vi "Trajectory_boom.vi"(0 "i":i32, 1 "if p2p":bool, 2 "ifSin?":bool, 3 "Target_Angle":dbl, 4 "if end8":bool, 5 "q":dbl[](array[numeric]), 7 "qd":dbl[](array[numeric]), 9 "qdd":dbl[](array[numeric]), 10 "if  Ramp":bool, 11 "qddd":dbl[](array[numeric]), 12 "qd8_1":dbl[](array[numeric]), 13 "qd8_dot_2":dbl[](array[numeric]), 14 "qd8_ddot_2":dbl[](array[numeric])) -> (6 "qd1_tol":dbl[](array[numeric]))   [LabVIEW 2020]
uses:
  <vilib>/imath/engines/lvmath2/RunTimeEngine/Managers/WorkSpace/UID Generator.vi
  <vilib>/imath/engines/lvmath2/RunTimeEngine/RunTimeType/NIMS_RunTimeType_From StrictType (excl LVString).vi
  <instcachedir>/0/NIMS_RunTimeType_From StrictType (excl LVString)_283B1B2000484AAA8744D21CE97EA49F.lvgen/NIMS_RunTimeType_From StrictType (excl LVString)_283B1B2000484AAA8744D21CE97EA49F_000.vi
  <vilib>/imath/engines/lvmath2/RunTimeEngine/LocalVariableDefStatement/MC_LocalVariableDefStatement_Display.vi
  <vilib>/imath/engines/lvmath2/RunTimeEngine/Managers/SymbolTable/Clear UID.vi
  <vilib>/imath/engines/lvmath2/RunTimeEngine/NodeEndStatement/NIMS_NodeEndStatement_Output.vi
  <instcachedir>/0/NIMS_NodeEndStatement_Output_53EC0D466D134D7ABD903AC30B43404B.lvgen/NIMS_NodeEndStatement_Output_53EC0D466D134D7ABD903AC30B43404B_001.vi
  <vilib>/imath/engines/lvmath2/RunTimeEngine/ErrorHandling/NIMS_Finalize Error.vi
  <vilib>/imath/engines/lvmath2/RunTimeEngine/VariableToken/NIMS_VariableToken_CondDefined.vi
  <instcachedir>/0/NIMS_VariableToken_CondDefined_537E119D71C74F9D9452D6FF923F1E1F.lvgen/NIMS_VariableToken_CondDefined_537E119D71C74F9D9452D6FF923F1E1F_003.vi
  <vilib>/imathl/engines/lvmath/Functions/Error Handling/Create Error.vi
  <instcachedir>/0/NIMS_VariableToken_CondDefined_537E119D71C74F9D9452D6FF923F1E1F.lvgen/NIMS_VariableToken_CondDefined_537E119D71C74F9D9452D6FF923F1E1F_005.vi
  <vilib>/imath/engines/lvmath/Functions/Error Handling/MergeErrorsWrapper.vi
  <instcachedir>/0/NIMS_NodeEndStatement_Output_53EC0D466D134D7ABD903AC30B43404B.lvgen/NIMS_NodeEndStatement_Output_53EC0D466D134D7ABD903AC30B43404B_010.vi
  <instcachedir>/0/NIMS_NodeEndStatement_Output_53EC0D466D134D7ABD903AC30B43404B.lvgen/NIMS_NodeEndStatement_Output_53EC0D466D134D7ABD903AC30B43404B_005.vi
  <vilib>/imath/engines/lvmath2/RunTimeEngine/Managers/SymbolTable/NIMS_WorkSpace.lvlib
panel:
  out "AlphaWF":dbl
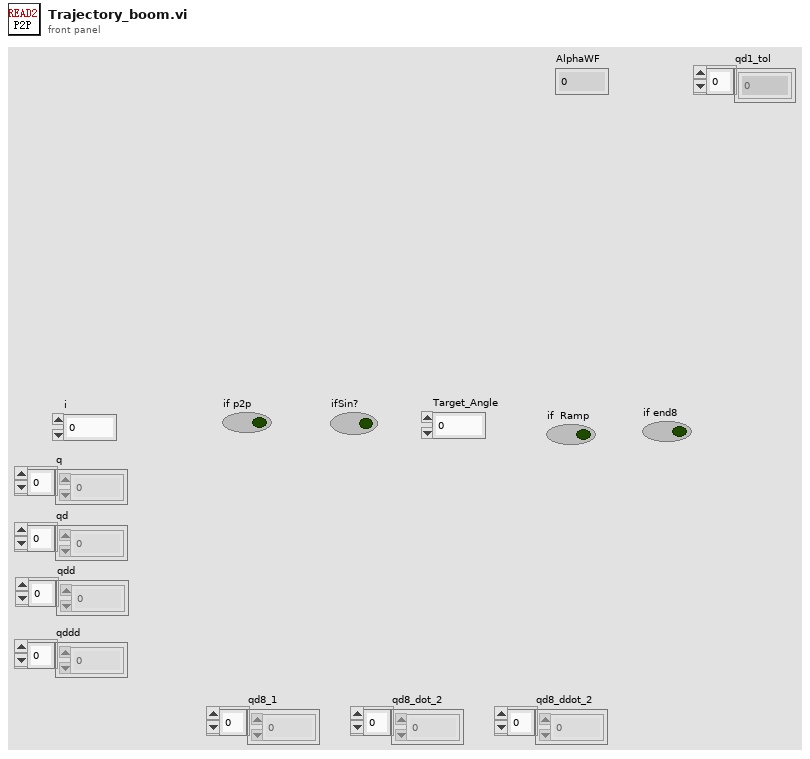
[diagram p1: front panel]
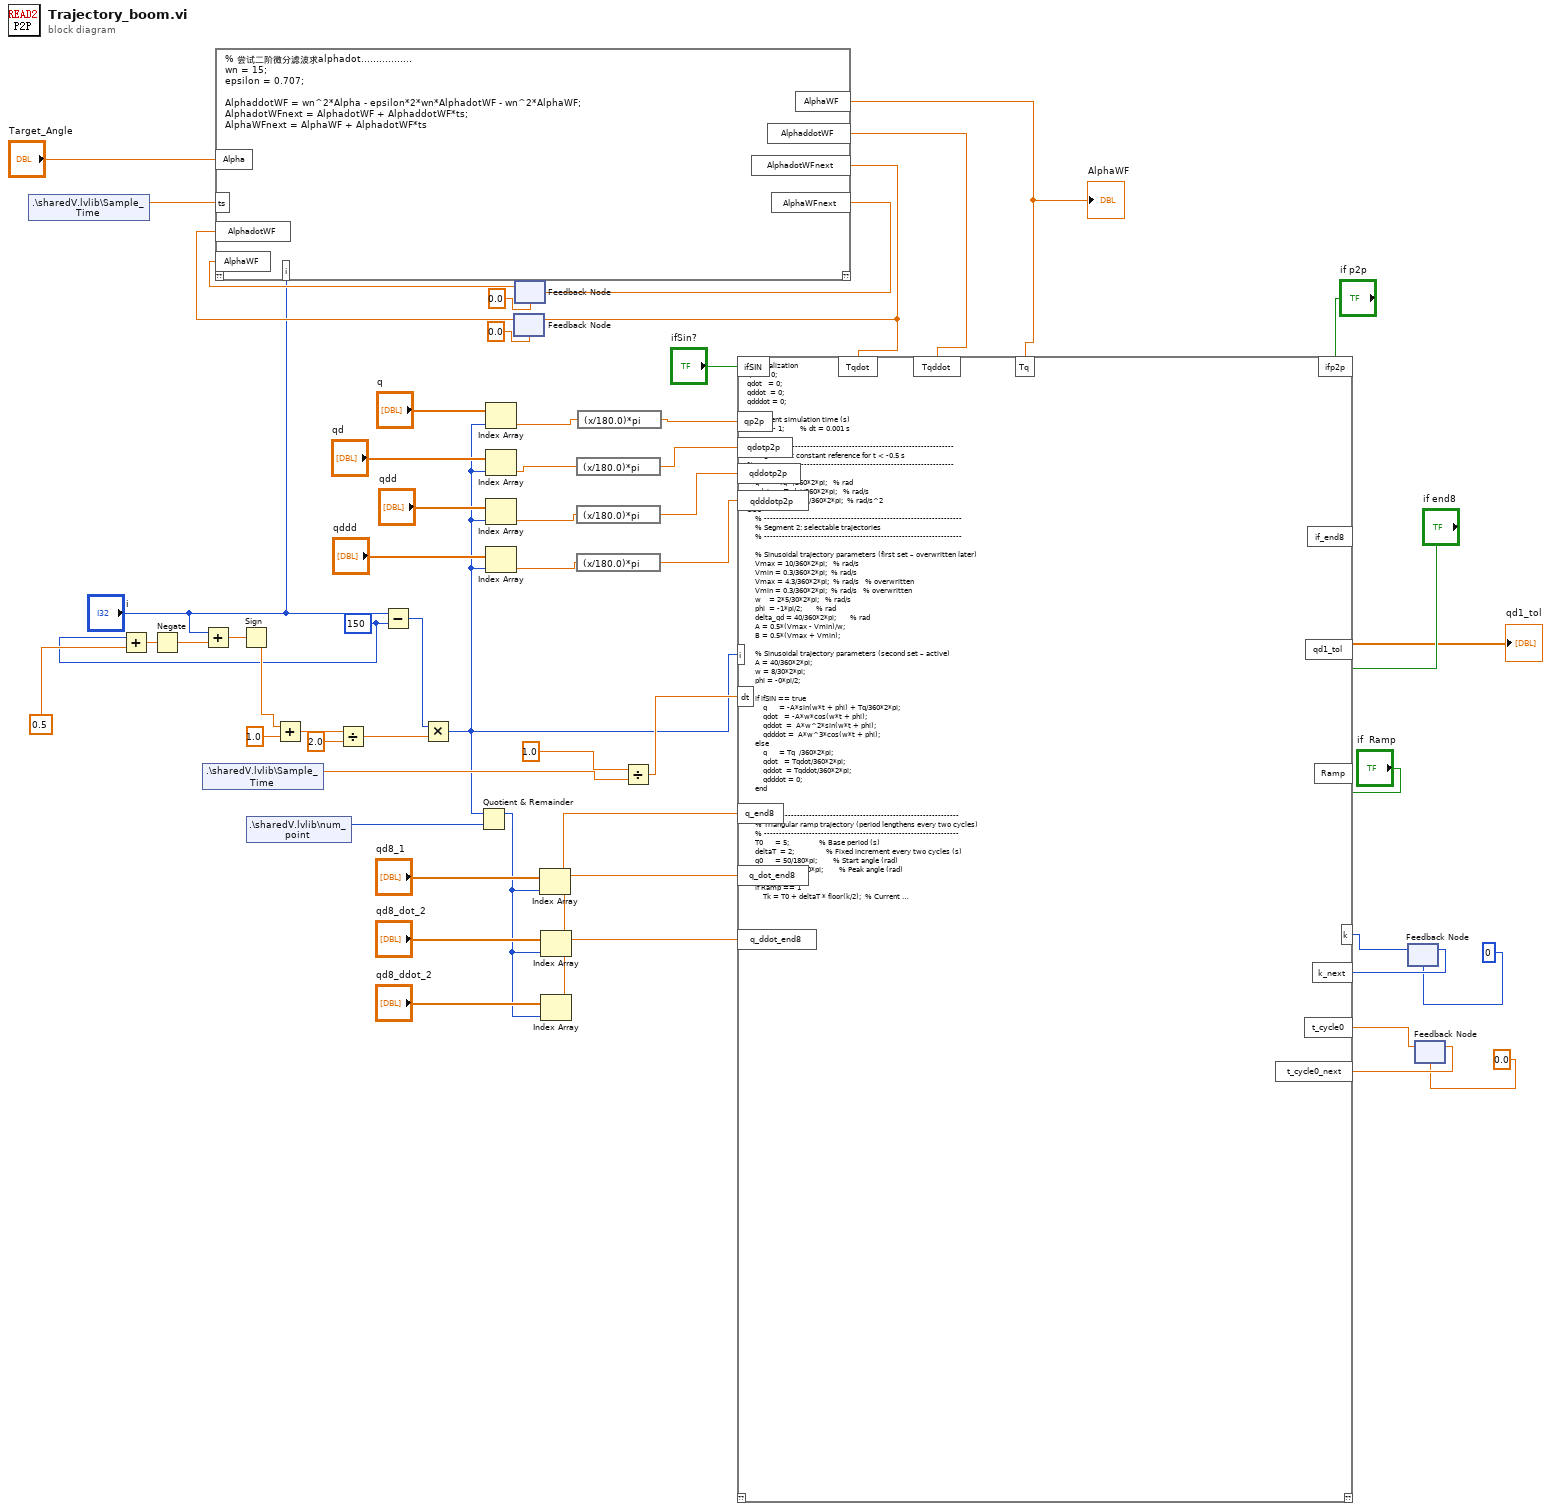
[diagram p0: block diagram]
diagram:
  w31 = 150 ("y")
  n1 = shared-variable ".\\sharedV.lvlib\\Sample_Time"() -> (w45:dbl)  [unwired: 1 in, 1 out]
  n2 = Add(x=w31, y=0.5) -> (x+y=w32:dbl)
  n3 = Negate(x=w32) -> (-x=w41:dbl)
  n4 = Add(x="i", y=w41) -> (x+y=w40:dbl)
  n5 = shared-variable ".\\sharedV.lvlib\\Sample_Time"() -> (w43:dbl)  [unwired: 1 in, 1 out]
  n6 = Sign(1:w40) -> (0:w38:dbl)
  n7 = shared-variable ".\\sharedV.lvlib\\num_point"() -> (w23:i32)  [unwired: 1 in, 1 out]
  n8 = Add(x=w38, y=1.0) -> (x+y=w36:dbl)
  n9 = Divide(x=w36, y=2.0) -> (x/y=w35:dbl)
  n10 = Subtract(x="i", y=w31) -> (x-y=w34:i32)
  n11 = Multiply(x=w34, y=w35) -> (x*y=w20:i32)
  n12 = Quotient & Remainder(x=w20, y=w23) -> (x-y*floor(x/y)=w22:i32)  [unwired: 1 out]
  n13 = Index Array(array="q", index=w20) -> (element=w12:dbl)
  n14 = Index Array(array="qd", index=w20) -> (element=w14:dbl)
  n15 = Index Array(array="qdd", index=w20) -> (element=w17:dbl)
  n16 = Index Array(array="qddd", index=w20) -> (element=w18:dbl)
  n17 = feedback #1(0.0 ("AlphadotWFnext")) -> (w47:dbl)
  n18 = feedback #2(0.0 ("AlphaWFnext")) -> (w49:dbl)
  n19 = mathscript code="% 尝试二阶微分滤波求alphadot.................\nwn = 15;\nepsilon = 0.707;\n\nAlphaddotWF = wn^2*Alpha - epsilon*2*wn*AlphadotWF - wn^2*AlphaWF;\nAlphadotWFnext = AlphadotWF + AlphaddotWF*ts;\nAlphaWFnext = AlphaWF + AlphadotWF*ts"("AlphaWF"=w49, "ts"=w45, "AlphadotWF"=w47, "Alpha"="Target_Angle", "i"="i") -> ("AlphaWFnext"=w50:dbl, "AlphadotWFnext"=w8:dbl, "AlphaWF"=w10:dbl, "AlphaddotWF"=w9:dbl)  [unwired: 1 in, 1 out]
  "AlphaWF" <- w10
  n20 = feedback-in #1(w8) -> ()
  n21 = feedback-in #2(w50) -> ()
  n22 = Index Array(array="qd8_1", index=w22) -> (element=w26:dbl)
  n23 = Index Array(array="qd8_dot_2", index=w22) -> (element=w25:dbl)
  n24 = Index Array(array="qd8_ddot_2", index=w22) -> (element=w24:dbl)
  n25 = expression code="(x/180.0)*pi" ("角度转换至弧度")(w14) -> (w15:dbl)
  n26 = expression code="(x/180.0)*pi" ("角度转换至弧度")(w17) -> (w16:dbl)
  n27 = expression code="(x/180.0)*pi" ("角度转换至弧度")(w18) -> (w19:dbl)
  n28 = expression code="(x/180.0)*pi" ("角度转换至弧度")(w12) -> (w13:dbl)
  n29 = Divide(x=1.0, y=w43) -> (x/y=w42:dbl)
  n30 = feedback #3(0) -> (w5:i32)
  n31 = feedback #4(0.0 ("AlphadotWFnext")) -> (w3:dbl)
  n32 = mathscript code="% Initialization\nq      = 0;\nqdot   = 0;\nqddot  = 0;\nqdddot = 0;\n\n% Current simulation time (s)\nt = i/dt - 1;        % dt = 0.001 s\n\n% ------------------------------------------------------------------\n% Segment 1: constant reference for t < -0.5 s\n% ------------------------------------------------------------------\nif t < -0.5\n    q      = Tq   /360*2*pi;   % rad\n    qdot   = Tqdot/360*2*pi;   % rad/s\n    qddot  = Tqddot/360*2*pi;  % rad/s^2\nelse\n    % ------------------------------------------------------------------\n    % Segment 2: selectable trajectories\n    % ------------------------------------------------------------------\n\n    % Sinusoidal trajectory parameters (first set – overwritten later)\n    Vmax = 10/360*2*pi;   % rad/s\n    Vmin = 0.3/360*2*pi;  % rad/s\n    Vmax = 4.3/360*2*pi;  % rad/s   % overwritten\n    Vmin = 0.3/360*2*pi;  % rad/s   % overwritten\n    w    = 2*5/30*2*pi;   % rad/s\n    phi  = -1*pi/2;       % rad\n    delta_qd = 40/360*2*pi;       % rad\n    A = 0.5*(Vmax - Vmin)/w;\n    B = 0.5*(Vmax + Vmin);\n\n    % Sinusoidal trajectory parameters (second set – active)\n    A = 40/360*2*pi;\n    w = 8/30*2*pi;\n    phi = -0*pi/2;\n\n    if ifSIN == true\n        q      = -A*sin(w*t + phi) + Tq/360*2*pi;\n        qdot   = -A*w*cos(w*t + phi);\n        qddot  =  A*w^2*sin(w*t + phi);\n        qdddot =  A*w^3*cos(w*t + phi);\n    else\n        q      = Tq  /360*2*pi;\n        qdot   = Tqdot/360*2*pi;\n        qddot  = Tqddot/360*2*pi;\n        qdddot = 0;\n    end\n     \n\n    % -----------------------------------------------------------------\n    % Triangular ramp trajectory (period lengthens every two cycles)\n    % -----------------------------------------------------------------\n    T0      = 5;               % Base period (s)\n    deltaT  = 2;                % Fixed increment every two cycles (s)\n    q0      = 50/180*pi;        % Start angle (rad)\n    qPeak   = 80/180*pi;        % Peak angle (rad)\n \n    if Ramp == 1\n        Tk = T0 + deltaT * floor(k/2);  % Current period length\n\n        % Move to next cycle when time exceeds current period\n        if t >= t_cycle0 + Tk\n            t_cycle0 = t_cycle0 + Tk;\n            k        = k + 1;\n            Tk       = T0 + deltaT * floor(k/2);\n        end\n\n        tau = t - t_cycle0;             % Relative time within cycle\n\n        % Triangular wave\n        TkHalf = Tk / 2;\n        if tau <= TkHalf\n            q_ramp = q0 + (qPeak - q0) * (tau / TkHalf);\n        else\n            q_ramp = qPeak - (qPeak - q0) * ((tau - TkHalf) / TkHalf);\n        end\n       t_cycle0_next = t_cycle0;\n       k_next = k;\n        \n    end\n     if Ramp == 1\n         q      = q_ramp;\n         qdot   = 0;\n         qddot  = 0;\n         qdddot = 0;\n     end\n\n    % ------------------------------------------------------------------\n    % End-point set-point override\n    % ------------------------------------------------------------------\n    if if_end8 == true\n        q      = q_end8;\n        qdot   = q_dot_end8;\n        qddot  = q_ddot_end8;\n        qdddot = 0;\n    end\n\n    % ------------------------------------------------------------------\n    % Point-to-point trajectory override\n    % ------------------------------------------------------------------\n    if ifp2p == 1\n        q      = qp2p;\n        qdot   = qdotp2p;\n        qddot  = qddotp2p;\n        qdddot = qdddotp2p;\n    end\n\n\nend\n\n% Output vector [position; velocity; acceleration; jerk]\nqd1_tol = [q; qdot; qddot; qdddot];"("ifSIN"="ifSin?", "qp2p"=w13, "qdotp2p"=w15, "qddotp2p"=w16, "qdddotp2p"=w19, "i"=w20, "ifp2p"="if p2p", "Tq"=w10, "Tqdot"=w8, "Tqddot"=w9, "dt"=w42, "q_end8"=w26, "q_dot_end8"=w25, "q_ddot_end8"=w24, "if_end8"="if end8", "Ramp"="if  Ramp", "k"=w5, "t_cycle0"=w3) -> ("qd1_tol"=→"qd1_tol":dbl[], "k_next"=w6:i32, "t_cycle0_next"=w4:dbl)  [unwired: 1 in, 1 out]
  n33 = feedback-in #3(w6) -> ()
  n34 = feedback-in #4(w4) -> ()
